vi "Wait-for-new-image.vi"(6 "Index in":i32=1000, 8 "error in":errorcluster, 9 "Acq. stats in":T1, 10 "Buffer element in":T2 {"Temperature characteristics"."Stand. dev. temperature" format="%#.1f"; "Temperature characteristics"."Min. temperature" format="%#.0f"; "Temperature characteristics"."Max. temperature" format="%#.0f"; "Temperature characteristics"."Average temperature" format="%#.0f"}, 11 "Buffers in":refnum<class "CV-Buffers.lvclass">) -> (0 "error IO":errorcluster, 1 "Acq. stats":T1, 2 "Buffer element":T2 {"Temperature characteristics"."Stand. dev. temperature" format="%#.1f"; "Temperature characteristics"."Min. temperature" format="%#.0f"; "Temperature characteristics"."Max. temperature" format="%#.0f"; "Temperature characteristics"."Average temperature" format="%#.0f"}, 3 "Buffers":refnum<class "CV-Buffers.lvclass">, 4 "Index":i32, 5 "New data?":bool)   [LabVIEW 2013, in "CameraVision.lvlib" / "CV-Main.lvclass"]
uses:
  CV-Main.lvclass
  Buffers/CV-Buffers.lvclass
  Acquisition/Acquisition-stats.ctl
  Buffers/Storage-buffer.ctl
  <vilib>/vision/Image Controls.llb/IMAQ Image.ctl
  Temperature/Temperature-characteristics.ctl
  Analysis/Characteristics-cluster.ctl
  Buffers/CV-Buffers.lvclass/CV-Buffers.ctl
  Buffers/Read Processing buffer.vi
  Acquisition/CV-Acquisition.lvclass
  Temperature/CV-Temperature.lvclass
  Analysis/CV-Analysis.lvclass
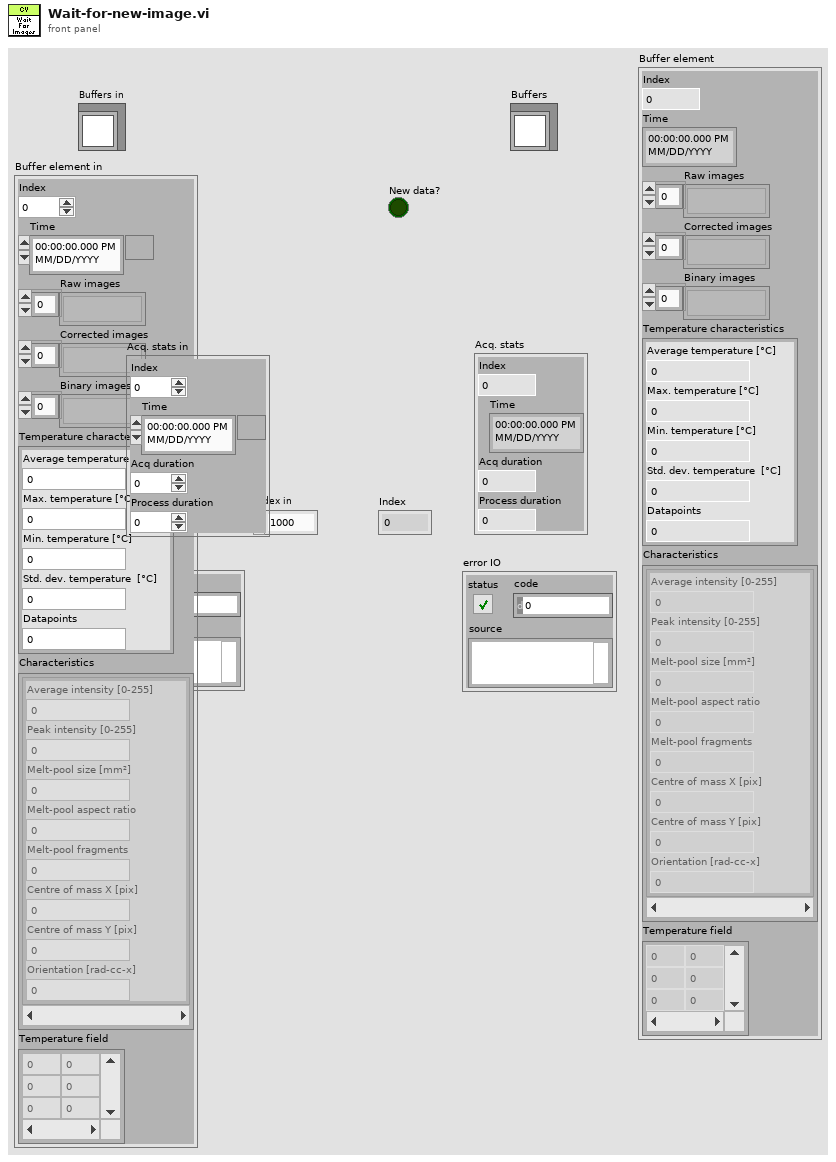
[diagram p1: front panel]
types:
  T1 = typedef "CameraVision.lvlib/CV-Acquisition.lvclass/Acquisition-stats.ctl" = cluster{"Index":i32, "Time":timestamp, "Acq duration":dbl, "Process duration":dbl}
  T2 = typedef "CameraVision.lvlib/CV-Buffers.lvclass/Storage-buffer.ctl" = cluster{"Index":i32, "Time":timestamp, "Raw images":T3[], "Corrected images":T3[], "Binary images":T3[], "Temperature characteristics":T4, "Characteristics":T5[], "Temperature field":dbl[][]}
  T3 = typedef "IMAQ Image.ctl" = refnum<image>
  T4 = typedef "CameraVision.lvlib/CV-Temperature.lvclass/Temperature-characteristics.ctl" = cluster{"Average temperature ":dbl, "Max. temperature":dbl, "Min. temperature":dbl, "Stand. dev. temperature":dbl, "Datapoints":dbl}
  T5 = typedef "CameraVision.lvlib/CV-Analysis.lvclass/Characteristics-cluster.ctl" = cluster{"Average intensity":dbl, "Peak intensity":dbl, "Melt-pool size":dbl, "Melt-pool aspect ratio":dbl, "Melt-pool fragments":dbl, "Centre of mass X":dbl, "Centre of mass Y":dbl, "Orientation":dbl}
  T6 = typedef "CameraVision.lvlib/CV-Buffers.lvclass/Storage-buffer-refs.ctl" = cluster{"Raw images":T3[], "Corrected images":T3[], "Binary images":T3[]}
  T7 = typedef "CameraVision.lvlib/Buffers.lvclass/Processing-buffer.ctl" = cluster{"Index":i32, "Time":timestamp, "Raw images":T3[]}
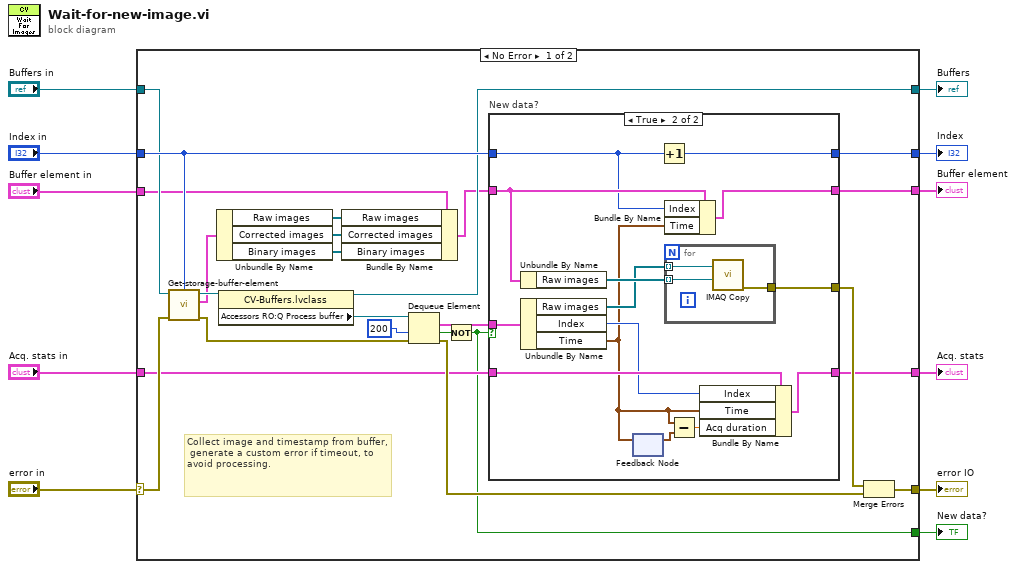
[diagram p0: block diagram]
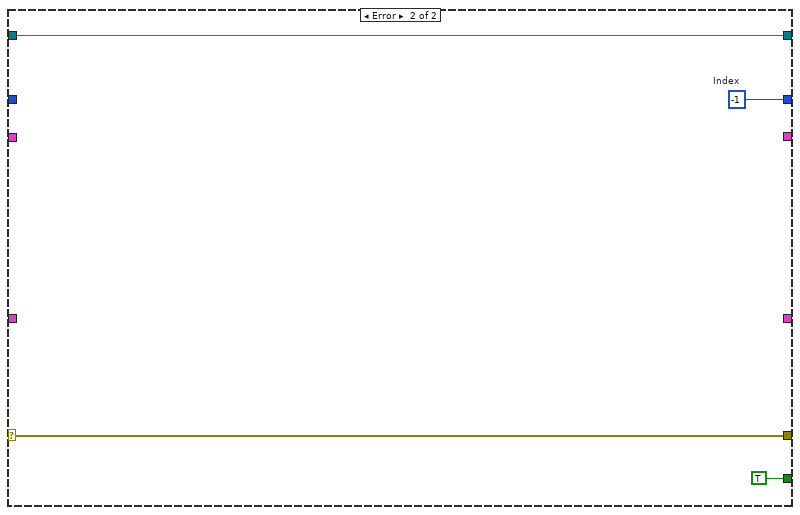
[diagram p3: hidden frame]
diagram:
  n1 = case shown="No Error" "error in" {
    selector: "error in" -> [w28 w59]
    tunnel: [w23 w59] -> w11
    tunnel: "Buffers in" -> [w29 w56]
    tunnel: "Index in" -> [w30 _]
    tunnel: [w32 w58] -> w7
    tunnel: [w25 _] -> w6
    tunnel: [w24 _] -> w3
    tunnel: [w12 TRUE ("timed out?")] -> w5
    tunnel: [w20 w56] -> w4
    tunnel: "Buffer element in" -> [w14 _]
    tunnel: "Acq. stats in" -> [w13 _]
    frame No Error {
      # "Collect image and timestamp from buffer,\n generate a custom error if timeout, to \navoid processing."
      n2 = call "Get-storage-buffer-element.vi"("error in (no error)"=w28, "Index"=w30, "Buffers in"=w29) -> ("error out"=w27:errorcluster, "Element ref"=w19:T6, "Buffers out"=w26:refnum<class "CV-Buffers.lvclass">)  [unwired: 6 in]
      n3 = Unbundle By Name(w19) -> ("Raw images"=w18:T3[], "Corrected images"=w17:T3[], "Binary images"=w16:T3[])
      n4 = property class="CV-Buffers.lvclass"(reference=w26) -> (reference out=w20:refnum<class "CV-Buffers.lvclass">, "Accessors RO:Q Process buffer"=w34:refnum<queue>)  [unwired: 1 in, 1 out]
      n5 = Bundle By Name(cluster=w14, "Raw images"=w18, "Corrected images"=w17, "Binary images"=w16) -> (w15:T2)
      n6 = Dequeue Element(queue=w34, timeout in ms (-1)=200, error in (no error)=w27) -> (element=w33:T7, timed out?=w21:bool, error out=w22:errorcluster)  [unwired: 1 out]
      n7 = Not(x=w21) -> (.not. x?=w12:bool)
      n8 = case "New data?" shown="True" w12 {
        tunnel: w33 -> [_ w52]
        tunnel: [_ w51] -> w35
        tunnel: [w38 w40] -> w32
        tunnel: w30 -> [w38 w39]
        tunnel: w15 -> [w36 w43]
        tunnel: w13 -> [w37 w48]
        tunnel: [w37 w44] -> w25
        tunnel: [w36 w42] -> w24
        frame False {
        }
        frame True {
          n9 = Unbundle By Name(w43) -> ("Raw images"=w50:T3[])
          n10 = Unbundle By Name(w52) -> ("Raw images"=w49:T3[], "Index"=w47:i32, "Time"=w41:timestamp)
          n11 = feedback-in #1(w41) -> ()
          n12 = feedback #1() -> (w45:timestamp)  [unwired: 1 in]
          n13 = Increment(x=w39) -> (x+1=w40:i32)
          n14 = Bundle By Name(cluster=w43, "Index"=w39, "Time"=w41) -> (w42:T2)
          n15 = for {
            tunnel: [w55] -> w51
            tunnel: w50 -> [w54] mode=indexing
            tunnel: w49 -> [w53] mode=indexing
            n16 = call "IMAQ Copy"("Image Dst"=w54, "Image Src"=w53) -> ("error out"=w55:errorcluster)  [unwired: 4 in, 1 out]
          }
          n17 = Subtract(x=w41, y=w45) -> (x-y=w46:dbl)
          n18 = Bundle By Name(cluster=w48, "Index"=w47, "Time"=w41, "Acq duration"=w46) -> (w44:T1)
        }
      }
      n19 = Merge Errors(w35, w22) -> (w23:errorcluster)
    }
    frame Error {
      w58 = -1  # Index
    }
  }
  "error IO" <- w11
  "Index" <- w7
  "Acq. stats" <- w6
  "New data?" <- w5
  "Buffers" <- w4
  "Buffer element" <- w3
